vi "Align TDMS File with Hard Disk Sector.vi"() -> ()   [LabVIEW 2023]
doc: "This example demonstrates how to align the header part of a .tdms file with integer multiples of 4 KB. This alignment is necessary if you want to use the Advanced TDMS VIs and functions to perform high-speed, unbuffered reading operations on the file."
uses:
  <vilib>/Utility/TDMS File Viewer/NI_TDMS File Viewer.lvlib
panel:
  out "converted successfully?":bool
  # "Overview: Demonstrates how to align the header part of a .tdms file with integer multiples of 4 KB. \nInstructions:\n1. Run the VI.\n2. Delete the .tdms file (located at [LabVIEW Data]\\Example Aligned.tdms) when you are done."
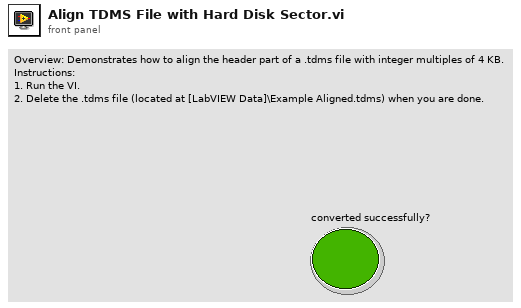
[diagram p1: front panel]
types:
  T1 = enum16{"open", "open or create", "create or replace", "create", "open (read-only)"}
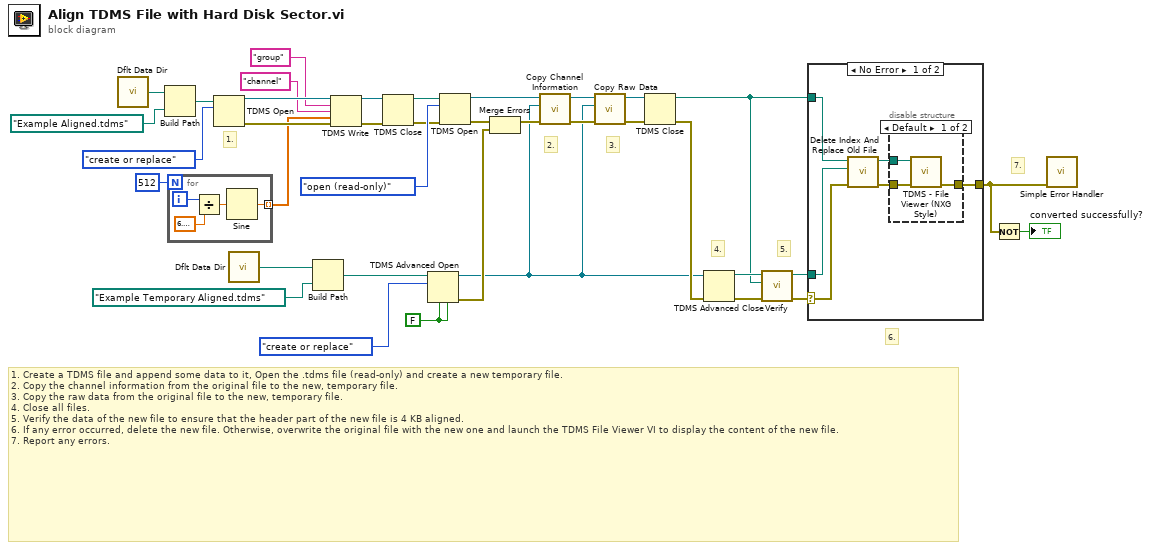
[diagram p0: block diagram]
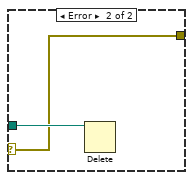
[diagram p3: hidden frame]
diagram:
  w35 = FALSE ("disable buffering? (T)")
  # "6."
  # "5."
  # "2."
  # "1."
  # "4."
  # "7."
  # "3."
  # "1. Create a TDMS file and append some data to it, Open the .tdms file (read-only) and create a new temporary file.\n2. Copy the channel information from the original file to the new, temporary file. \n3. Copy the raw data from the original file to the new, temporary file.\n4. Close all files.\n5. Verify the data of the new file to ensure that the header part of the new file is 4 KB aligned.\n6. If any error occurred, delete the new file. Otherwise, overwrite the original file with the new one and launch the TDMS File Viewer VI to display the content of the new file.\n7. Report any errors."
  n1 = call <vilib>:"Dflt Data Dir.vi"() -> ("App:Default Data Directory"=w12:path)
  n2 = Build Path(base path=w12, name or relative path=path "Example Aligned.tdms") -> (appended path=w11:path)
  n3 = for {
    N: 512 ("dimension size") -> [_]
    tunnel: [w41] -> w1 mode=indexing
    i -> [w40]
    n4 = Divide(x=w40, y=6.283185307179586) -> (x/y=w39:dbl)
    n5 = Sine(x=w39) -> (sin(x)=w41:dbl)
  }
  n6 = TDMS Open(10:T1."create or replace" ("operation (0:open)"), 11:w11) -> (0:w15:errorcluster, 3:w16:refnum<k34>)  [unwired: 5 in]
  n7 = call <vilib>:"Dflt Data Dir.vi"() -> ("App:Default Data Directory"=w3:path)
  n8 = Build Path(base path=w3, name or relative path=path "Example Temporary Aligned.tdms") -> (appended path=w34:path)
  n9 = TDMS Write(0:w16, 5:"group" ("group name in (Untitled)"), 7:"channel" ("group name in (Untitled)"), 9:w1, 11:w15) -> (4:w17:refnum<k34>, 15:w14:errorcluster)  [unwired: 1 in, 2 out]
  n10 = TDMS Close(8:w14, 11:w17) -> (0:w9:errorcluster, 3:w10:path)
  n11 = TDMS Advanced Open(4:w35, 6:w35, 10:T1."create or replace" ("operation (0:open)"), 11:w34) -> (0:w32:errorcluster, 3:w4:refnum<k34>)  [unwired: 1 in, 1 out]
  n12 = TDMS Open(8:w9, 10:T1."open (read-only)" ("operation"), 11:w10) -> (0:w28:errorcluster, 3:w27:refnum<k34>)  [unwired: 4 in]
  n13 = Merge Errors(w28, w32) -> (w33:errorcluster)
  n14 = call "Copy Channel Information.vi"("error in (no error)"=w33, "new tdms file"=w4, "original tdms file"=w27) -> ("error out"=w25:errorcluster, "dup original tdms file"=w26:refnum<k34>)  [unwired: 7 in]
  n15 = call "Copy Raw Data.vi"("error in (no error)"=w25, "new tdms file"=w4, "original tdms file"=w26) -> ("error out"=w20:errorcluster, "dup original tdms file"=w31:refnum<k34>)  [unwired: 7 in]
  n16 = TDMS Close(8:w20, 11:w31) -> (0:w24:errorcluster, 3:w21:path)
  n17 = TDMS Advanced Close(8:w24, 11:w4) -> (0:w23:errorcluster, 3:w22:path)  [unwired: 2 in]
  n18 = call "Verify.vi"("error in"=w23, "original file path"=w21, "new file path"=w22) -> ("error out"=w29:errorcluster, "new file path out"=w30:path)  [unwired: 7 in]
  n19 = case shown="No Error" w29 {
    selector: w29 -> [w42 w51]
    tunnel: w30 -> [w43 w52]
    tunnel: [w45 w51] -> w5
    tunnel: w21 -> [w47 _]
    frame No Error {
      n20 = call "Delete Index And Replace Old File.vi"("error in (no error)"=w42, "new file path"=w43, "old file path"=w47) -> ("error out"=w44:errorcluster, "new path"=w46:path)  [unwired: 7 in]
      n21 = disable-structure shown="Default" {
        disable-tunnel: w46 -> [w50 _]
        disable-tunnel: w44 -> [w49 _]
        disable-tunnel: [w48 _] -> w45
        frame condition #0 (active) {
          n22 = call <vilib>:"TDMS - File Viewer (NXG Style).vi"("error in"=w49, "file in"=w50) -> ("error out"=w48:errorcluster)  [unwired: 8 in, 1 out]
        }
        frame condition #1 {
        }
      }
    }
    frame Error {
      n23 = Delete(path (use dialog)=w52) -> ()  [unwired: 4 in, 3 out]
    }
  }
  n24 = Not(x=w5) -> (.not. x?=→"converted successfully?":bool)
  n25 = call <vilib>:"Simple Error Handler.vi"("error in (no error)"=w5) -> ()  [unwired: 4 in, 5 out]
